vi "Teleop.vi"(10 "Match Info":T1={"Autonomous Elapsed Seconds"=0.0, "TeleOp Elapsed Seconds"=0.0, "Disabled Elapsed Seconds"=0.0, "Visited Autonomous"=FALSE, "Visited TeleOp"=FALSE, "Visited Disabled"=FALSE, "Autonomous Settings"={"Autonomous Style"=enum."Independent", "VI Refnum"=refnum}}, 11 "Call Context":T2) -> ()   [LabVIEW 2012]
doc: "This VI is called for each TeleOp packet received from the DS where the robot is not disabled. It is often used to read from the joysticks and update I/O or to update setpoints for timed control loops. It should complete and return within 20 milliseconds or it may miss DS packets."
uses:
  <vilib>/Rock Robotics/WPI/DriverStation/WPI_DriverStationDerivedRobotMode.ctl
  <vilib>/Rock Robotics/WPI/DriverStation/WPI_DriverStationMatch Info.ctl
  Robot Global Data.vi
  <vilib>/Rock Robotics/Network Tables/SD Write Boolean.vi
  <vilib>/Rock Robotics/WPI/Joystick/WPI_JoystickGetSetRefNum.vi
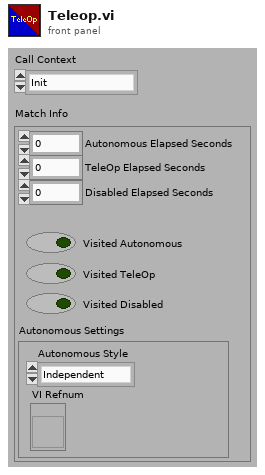
[diagram p1: front panel]
types:
  T1 = typedef "WPI_DriverStationMatch Info.ctl" = cluster{"Autonomous Elapsed Seconds":dbl, "TeleOp Elapsed Seconds":dbl, "Disabled Elapsed Seconds":dbl, "Visited Autonomous":bool, "Visited TeleOp":bool, "Visited Disabled":bool, "Autonomous Settings":cluster{"Autonomous Style":enum16{"Iterative", "Independent"}, "VI Refnum":refnum<vi>}}
  T2 = typedef "WPI_DriverStationDerivedRobotMode.ctl" = enum16{"Init", "Execute", "Stop"}
  T3 = typedef "WPI_JoystickDevRef.ctl" = cluster{"Device":T4}
  T4 = typedef "WPI_JoystickDeviceEnum.ctl" = enum16{"USB 1", "USB 2", "USB 3", "USB 4", "Kinect 1", "Kinect 2"}
  T5 = typedef "WPI_JoystickButtonState.ctl" = cluster{"Button 1":bool, "Button 2":bool, "Button 3":bool, "Button 4":bool, "Button 5":bool, "Button 6":bool, "Button 7":bool, "Button 8":bool, "Button 9":bool, "Button 10":bool, "Button 11":bool, "Button 12":bool}
  T6 = cluster{"axis 1 (x)":dbl, "axis 2 (y)":dbl, "axis 3 (throttle)":dbl, "axis 4":dbl, "axis 5":dbl, "axis 6":dbl}
  T7 = enum16{"Off", "Close Pyramid 3pt", "Far Pyramid 3pt", "Feeder Shot", "UD Far 3pt Shot"}
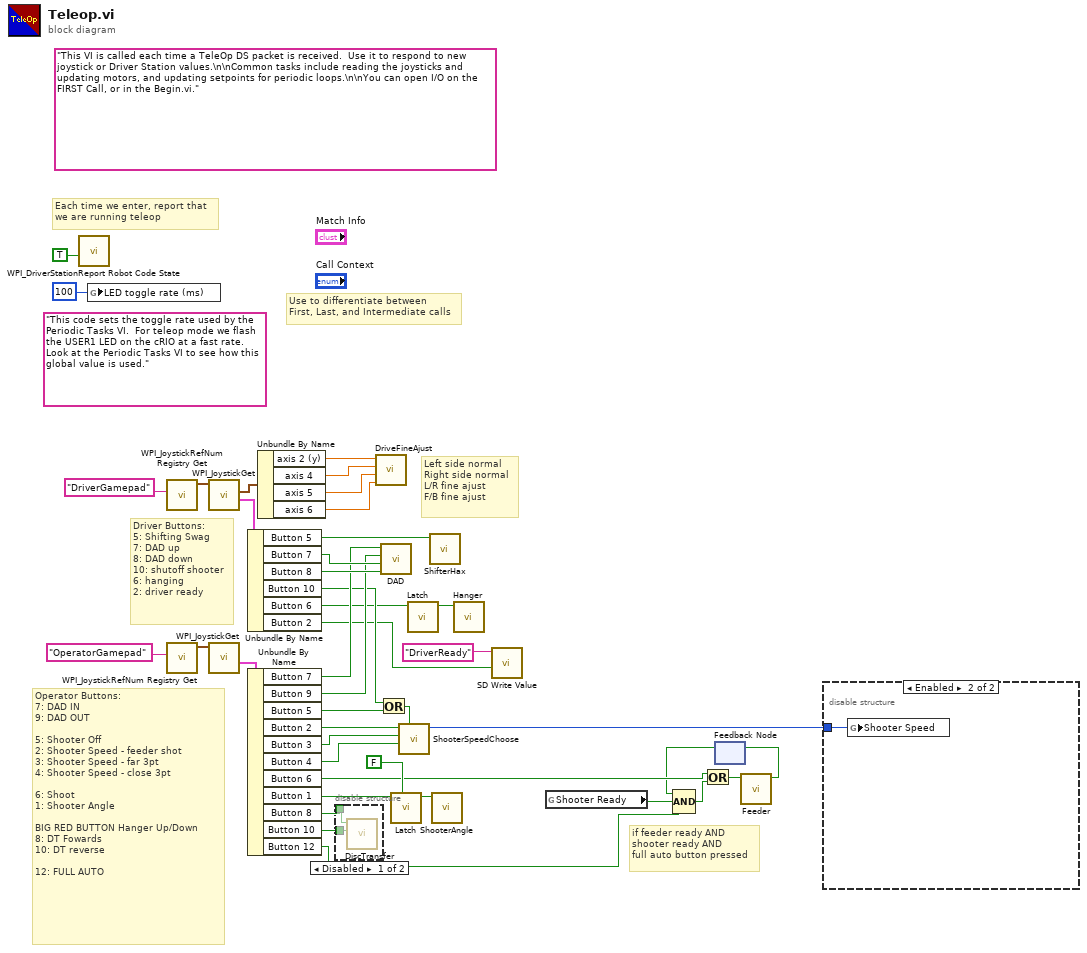
[diagram p0: block diagram]
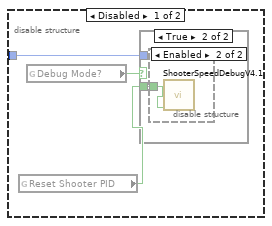
[diagram p2: hidden frame]
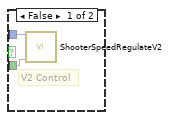
[diagram p3: hidden frame]
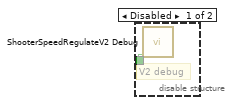
[diagram p4: hidden frame]
diagram:
  (unwired) "This code sets the toggle rate used by the Periodic Tasks VI.  For teleop mode we flash the USER1 LED on the cRIO at a fast rate.  Look at the Periodic Tasks VI to see how this global value is used."
  (unwired) "This VI is called each time a TeleOp DS packet is received.  Use it to respond to new joystick or Driver Station values.\n\nCommon tasks include reading the joysticks and updating motors, and updating setpoints for periodic loops.\n\nYou can open I/O on the FIRST Call, or in the Begin.vi."
  # "Left side normal\nRight side normal\nL/R fine ajust\nF/B fine ajust"
  # "if feeder ready AND\nshooter ready AND\nfull auto button pressed"
  # "Driver Buttons:\n5: Shifting Swag\n7: DAD up\n8: DAD down \n10: shutoff shooter\n6: hanging\n2: driver ready"
  # "Operator Buttons:\n7: DAD IN\n9: DAD OUT\n\n5: Shooter Off\n2: Shooter Speed - feeder shot\n3: Shooter Speed - far 3pt\n4: Shooter Speed - close 3pt\n\n6: Shoot\n1: Shooter Angle\n\nBIG RED BUTTON Hanger Up/Down\n8: DT Fowards\n10: DT reverse\n\n12: FULL AUTO"
  # "Each time we enter, report that\nwe are running teleop"
  # "Use to differentiate between\nFirst, Last, and Intermediate calls"
  n1 = call <vilib>:"WPI_DriverStationReport Robot Code State.vi"("TeleOp"=TRUE ("Autonomous")) -> ()  [unwired: 10 in, 1 out]
  n2 = global write "Robot Global Data.vi" "LED toggle rate (ms)"(u32 100 ("LED ms toggle rate")) -> ()
  n3 = call <vilib>:"WPI_JoystickRefNum Registry Get.vi"("refnum name"="DriverGamepad") -> ("JoystickDevRef"=w41:T3)  [unwired: 1 in, 9 out]
  n4 = call <vilib>:"WPI_JoystickRefNum Registry Get.vi"("refnum name"="OperatorGamepad") -> ("JoystickDevRef"=w36:T3)  [unwired: 1 in, 9 out]
  n5 = call <vilib>:"WPI_JoystickGet.vi"("JoystickDevRef"=w41) -> ("Buttons"=w37:T5, "Axes"=w38:T6)  [unwired: 1 in, 4 out]
  n6 = call <vilib>:"WPI_JoystickGet.vi"("JoystickDevRef"=w36) -> ("Buttons"=w35:T5)  [unwired: 1 in, 5 out]
  n7 = Unbundle By Name(w37) -> ("Button 5"=w32:bool, "Button 7"=w28:bool, "Button 8"=w27:bool, "Button 10"=w23:bool, "Button 6"=w21:bool, "Button 2"=w5:bool)
  n8 = Unbundle By Name(w35) -> ("Button 7"=w26:bool, "Button 9"=w25:bool, "Button 5"=w24:bool, "Button 2"=w18:bool, "Button 3"=w17:bool, "Button 4"=w16:bool, "Button 6"=w12:bool, "Button 1"=w22:bool, "Button 8"=w20:bool, "Button 10"=w19:bool, "Button 12"=w7:bool)
  n9 = Unbundle By Name(w38) -> ("axis 2 (y)"=w2:dbl, "axis 4"=w1:dbl, "axis 5"=w4:dbl, "axis 6"=w3:dbl)
  n10 = disable-structure shown="Disabled" {
    disable-tunnel: w20 -> [w43 _]
    disable-tunnel: w19 -> [w42 _]
    frame Disabled {
      n11 = call "DiscTransfer.vi"("DT Backwards"=w42, "DT Foward"=w43) -> ()  [unwired: 10 in]
    }
    frame Enabled {
    }
  }
  n12 = call "DriveFineAjust.vi"("Fine Ajust F/B"=w3, "Fine Ajust L/R"=w4, "Right Side Normal"=w1, "Left Side Normal"=w2) -> ()  [unwired: 8 in]
  n13 = Or(x=w23, y=w24) -> (x .or. y?=w15:bool)
  n14 = call "DAD.vi"("BAD DOWN"=w27, "BAD UP"=w28, "BAD OUT"=w25, "BAD IN"=w26) -> ()  [unwired: 7 in, 1 out]
  n15 = call "Latch.vi"("Default Value (false)"=FALSE, "Latch In"=w22) -> ("Latch Out"=w31:bool)  [unwired: 9 in]
  n16 = call "ShooterSpeedChoose.vi"("Shooter OFF"=w15, "Close 3pt Shot Button"=w16, "Far 3pt Shot Button"=w17, "Feedershot Button"=w18) -> ("Shooter Speed"=w34:T7)  [unwired: 7 in]
  n17 = call "Latch.vi"("Latch In"=w21) -> ("Latch Out"=w33:bool)  [unwired: 10 in]
  n18 = call "ShifterHax.vi"("Shift low?"=w32) -> ()  [unwired: 11 in]
  n19 = call "ShooterAngle.vi"("Shooter Angle Up?"=w31) -> ()  [unwired: 10 in, 1 out]
  n20 = call "Hanger.vi"("Hanger Up"=w33) -> ()  [unwired: 10 in, 1 out]
  n21 = call-poly <vilib>:"SD Write Value.vi"("Boolean"=w5, "Name"="DriverReady") -> ()  [unwired: 8 in, 2 out]
  n22 = global read "Robot Global Data.vi" "Shooter Ready"() -> (w8:bool)
  n23 = feedback #1() -> (w9:bool)  [unwired: 1 in]
  n24 = Compound Arithmetic op=AND(w9, w8, w7) -> (w11:bool)
  n25 = Or(x=w12, y=w11) -> (x .or. y?=w13:bool)
  n26 = call "Feeder.vi"("SHOOT Button"=w13) -> ("Ready To Shoot?"=w10:bool)  [unwired: 10 in]
  n27 = feedback-in #1(w10) -> ()
  n28 = disable-structure shown="Enabled" {
    disable-tunnel: w34 -> [w46 w52]
    frame Disabled {
      n29 = global read "Robot Global Data.vi" "Reset Shooter PID"() -> (w44:bool)
      n30 = global read "Robot Global Data.vi" "Debug Mode?"() -> (w45:bool)
      n31 = case shown="True" w45 {
        tunnel: w46 -> [w48 _]
        tunnel: w44 -> [w47 w49]
        frame False {
          # "V2 Control"
          n32 = call "ShooterSpeedRegulateV2.vi"("Shooter Speed"=w48, "Reset Shooter PID"=w47) -> ()  [unwired: 12 in, 2 out]
        }
        frame True {
          n33 = disable-structure shown="Enabled" {
            disable-tunnel: w49 -> [w50 w51]
            frame Disabled {
              # "V2 debug"
              n34 = call "ShooterSpeedRegulateV2 Debug.vi"("Reset Shooter PID"=w50) -> ()  [unwired: 13 in, 2 out]
            }
            frame Enabled {
              n35 = call "ShooterSpeedDebugV4.1.vi"("Reset PID"=w51) -> ()  [unwired: 9 in, 2 out]
            }
          }
        }
      }
    }
    frame Enabled {
      n36 = global write "Robot Global Data.vi" "Shooter Speed"(w52) -> ()
    }
  }
